vi "Test Generate AO Waveforms.vi"(8 "error in (no error)":errorcluster, 11 "Generator in":refnum<class "Generator.lvclass">) -> (0 "error out":errorcluster)   [LabVIEW 2019, in "Generator.lvclass"]
uses:
  Generator.lvclass
  typedefs/AO.Channel.Function--Enum.ctl
  typedefs/AO.Channel--Cluster.ctl
  typedefs/AO.Channel--Cluster--Array.ctl
panel:
  in  "configuration.AO Channels":T1 {"Frequency" format="%.3g"; "Offset" min=0.0001 max=10000.0 format="%.3g"; "Amplitude" format="%5.2p"; "Channel" min=0 max=10 format="%5.2p"}
  out "Resets":i16(graph)
  out "Intensity Graph":dbl[][](graph)
  in  "milliseconds to wait":u32=10
  out "Updates":i32=36
  out "Waveform Graph":waveform(dbl)[](graph)
  in  "sampling":cluster{"Fs":dbl, "#s":i32}={"Fs"=55000.0, "#s"=8000} {"Fs" format="%#_13g"}
  in  "stop":bool
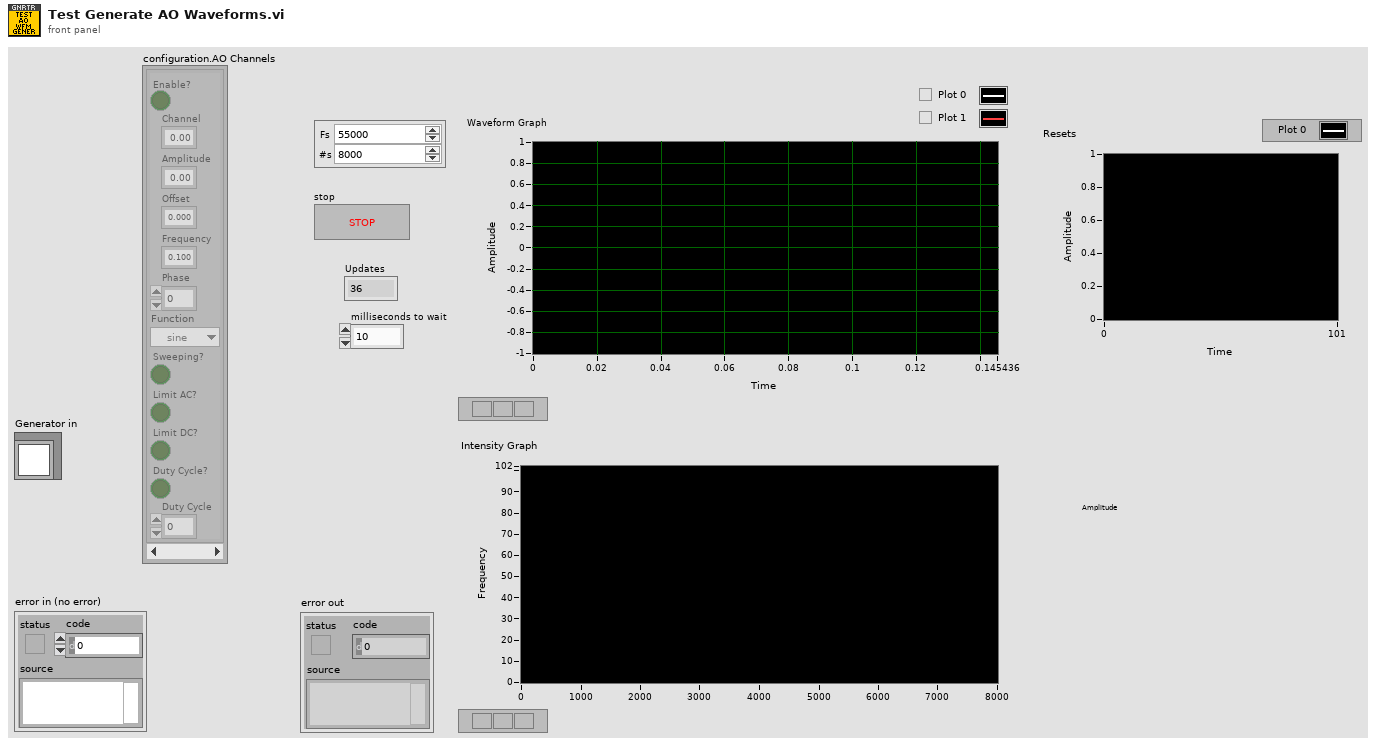
[diagram p1: front panel]
types:
  T1 = typedef "Generator.lvclass/AO.Channel--Cluster--Array.ctl" = T2[]
  T2 = typedef "Generator.lvclass/AO.Channel--Cluster.ctl" = cluster{"Enable?":bool, "Channel":i32, "Amplitude":dbl, "Offset":dbl, "Frequency":dbl, "Phase":dbl, "Function":T3, "Sweeping?":bool, "Limit AC?":bool, "Limit DC?":bool, "Duty Cycle?":bool, "Duty Cycle":dbl}
  T3 = typedef "Generator.lvclass/AO.Channel.Function--Enum.ctl" = enum16{"sine", "square", "triangle", "saw"}
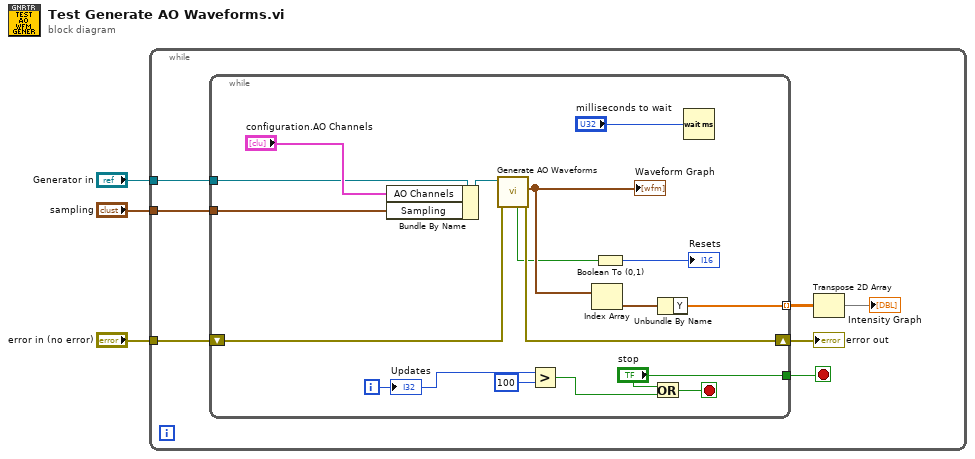
[diagram p0: block diagram]
diagram:
  n1 = while {
    tunnel: "error in (no error)" -> [w9]
    tunnel: "Generator in" -> [w6]
    tunnel: "sampling" -> [w5]
    stop <- w4 stop-if-true
    n2 = while {
      shift-right: [w25] -> w10
      shift-left: w9 -> [w26]
      tunnel: [w18] -> w8 mode=indexing
      tunnel: w6 -> [w14]
      tunnel: w5 -> [w12]
      tunnel: ["stop"] -> w4
      i -> [w24]
      stop <- w21 stop-if-true
      n3 = Bundle By Name(cluster=w14, "AO Channels"="configuration.AO Channels", "Sampling"=w12) -> (w13:refnum<class "Generator.lvclass">)
      n4 = call "Generate AO Waveforms.vi"("error in (no error)"=w26, "Generator in"=w13) -> ("error out"=w25:errorcluster, "AO Array"=w20:waveform(dbl)[], "phase reset"=w17:bool)  [unwired: 6 in, 1 out]
      "Waveform Graph" <- w20
      n5 = Greater?(x=w24, y=100) -> (0:w22:bool)
      n6 = Index Array(array=w20) -> (element=w19:waveform(dbl))  [unwired: 1 in]
      n7 = Boolean To (0,1)(Boolean=w17) -> (0, 1=→"Resets":i16)
      n8 = Or(x="stop", y=w22) -> (x .or. y?=w21:bool)
      n9 = Unbundle By Name(w19) -> ("Y"=w18:dbl[])
      n10 = Wait (ms)(milliseconds to wait="milliseconds to wait") -> ()  [unwired: 1 out]
      "Updates" <- w24
    }
    "error out" <- w10
    n11 = Transpose 2D Array(2D array=w8) -> (transposed array=→"Intensity Graph":dbl[][])
  }
